vi "rotate array.vi"(11 "Array 2":dbl[][](array[numeric])) -> (3 "Array":dbl[][](array[numeric]))   [LabVIEW 2012, in "BMC.lvclass"]
uses:
  BMC.lvclass
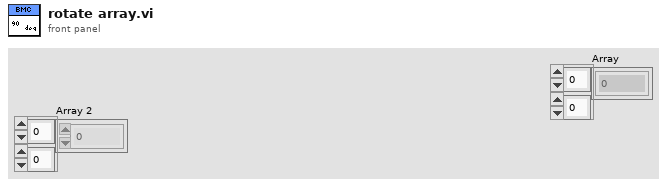
[diagram p1: front panel]
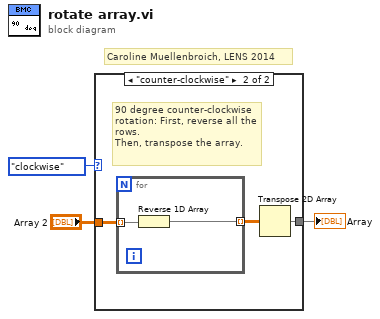
[diagram p0: block diagram]
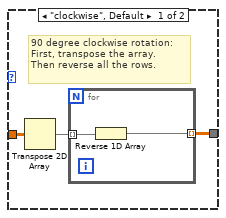
[diagram p2: hidden frame]
diagram:
  # "Caroline Muellenbroich, LENS 2014"
  n1 = case shown="\"counter-clockwise\"" enum16{"clockwise", "counter-clockwise"}."clockwise" ("Direction (clockwise)") {
    tunnel: "Array 2" -> [w4 w9]
    tunnel: [w5 w10] -> w2
    frame "clockwise", Default {
      # "90 degree clockwise rotation: First, transpose the array.\nThen reverse all the rows."
      n2 = Transpose 2D Array(2D array=w4) -> (transposed array=w6:dbl[][])
      n3 = for {
        tunnel: w6 -> [w8] mode=indexing
        tunnel: [w7] -> w5 mode=indexing
        n4 = Reverse 1D Array(array=w8) -> (reversed array=w7:dbl[])
      }
    }
    frame "counter-clockwise" {
      # "90 degree counter-clockwise rotation: First, reverse all the rows.\nThen, transpose the array."
      n5 = for {
        tunnel: w9 -> [w12] mode=indexing
        tunnel: [w13] -> w11 mode=indexing
        n6 = Reverse 1D Array(array=w12) -> (reversed array=w13:dbl[])
      }
      n7 = Transpose 2D Array(2D array=w11) -> (transposed array=w10:dbl[][])
    }
  }
  "Array" <- w2
